vi "Inspect Main.vi"() -> ()   [LabVIEW 2019]
uses:
  Inspect States.ctl
  Common.llb/IVB Global Variable Data Structure.ctl
  Common.llb/IVB Global Variable Type.ctl
  Common.llb/IVB Global Variable Data Type.ctl
  Common.llb/IVB State Machine Data.ctl
  Common.llb/IVB State Machine - States Array.ctl
  Common.llb/IVB State Machine - State.ctl
  Common.llb/IVB State Machine - Transitions Array.ctl
  Common.llb/IVB State Machine - Transition.ctl
  Common.llb/IVB State Machine - Free Labels Array.ctl
  Common.llb/IVB State Machine - Free Label.ctl
  Common.llb/IVB Custom UI - Data.ctl
  Common.llb/IVB Measure ID.ctl
  Common.llb/IVB Execution Function Code.ctl
  Common.llb/IVB VDM Palette Type.ctl
  Common.llb/IVB Decision Maker - Step Results AND Function.ctl
  <vilib>/Utility/sysdir.llb/System Directory Type.ctl
  Common.llb/IVB Results Manager Function.ctl
  Common.llb/IVB CoordSys Manager Function.ctl
  Common.llb/IVB ROI Manager Function.ctl
  Common.llb/IVB State Machine Data Manager Function.ctl
  Common.llb/IVB Palette Manager Function.ctl
  Common.llb/IVB Image Providers Manager Function.ctl
  Common.llb/IVB Global Variable - Manager Mode.ctl
  Common.llb/IVB Custom UI Manager Function.ctl
  Common.llb/IVB Codegen Globals.vi
  Common.llb/IVB Application Paths Global.vi
panel:
  in  "VBAI User Palettes Folder":string="National Instruments\\Vision Builder AI\\Palettes"
  in  "VBAI Flat Field Folder":string="National Instruments\\Vision Builder AI\\Flat Field"
  in  "VBAI Calibration Folder":string="National Instruments\\Vision Builder AI\\Calibration"
  in  "Custom UI Data":T1={"VI Path"=path "", "Use Custom UI"=FALSE, "Show Stats"=TRUE, "Show Table BG Color"=TRUE, "Auto Populate Table"=TRUE, "Table Measure IDs"=[{"Step GUID"="", "Result GUID"="{BE7D05E6-89B2-42AA-A48C-21281F1D1FF2}", "Index"=0}, {"Step GUID"="04378377", "Result GUID"="PASS/FAIL", "Index"=0}, {"Step GUID"="88198009", "Result GUID"="PASS/FAIL", "Index"=0}, {"Step GUID"="03525588", "Result GUID"="PASS/FAIL", "Index"=0}, {"Step GUID"="93671840", "Result GUID"="PASS/FAIL", "Index"=0}, {"Step GUID"="87659981", "Result GUID"="PASS/FAIL", "Index"=0}, {"Step GUID"="92409063", "Result GUID"="PASS/FAIL", "Index"=0}, {"Step GUID"="18845728", "Result GUID"="PASS/FAIL", "Index"=0}, {"Step GUID"="52930538", "Result GUID"="PASS/FAIL", "Index"=0}], "FP Width"=1007, "FP Height"=634, "Version"="6.1.0.0", "Strip Chart Data"={"Names"=[], "History Size"=[]}}
  in  "Inspection Name":string="LICENSE PLATE"
  in  "State Data":T3 {"Transitions"."Scale"."Y" format="%.2f"; "Transitions"."Scale"."X" format="%.2f"}
  out "Image":T10(plugin-control)
  in  "Global Variable Data":T11[](array[typedef])
  in  "Initial State":T14
  in  "Stop":bool
  out "Pass Fail":bool=TRUE caption="Inspection Status"
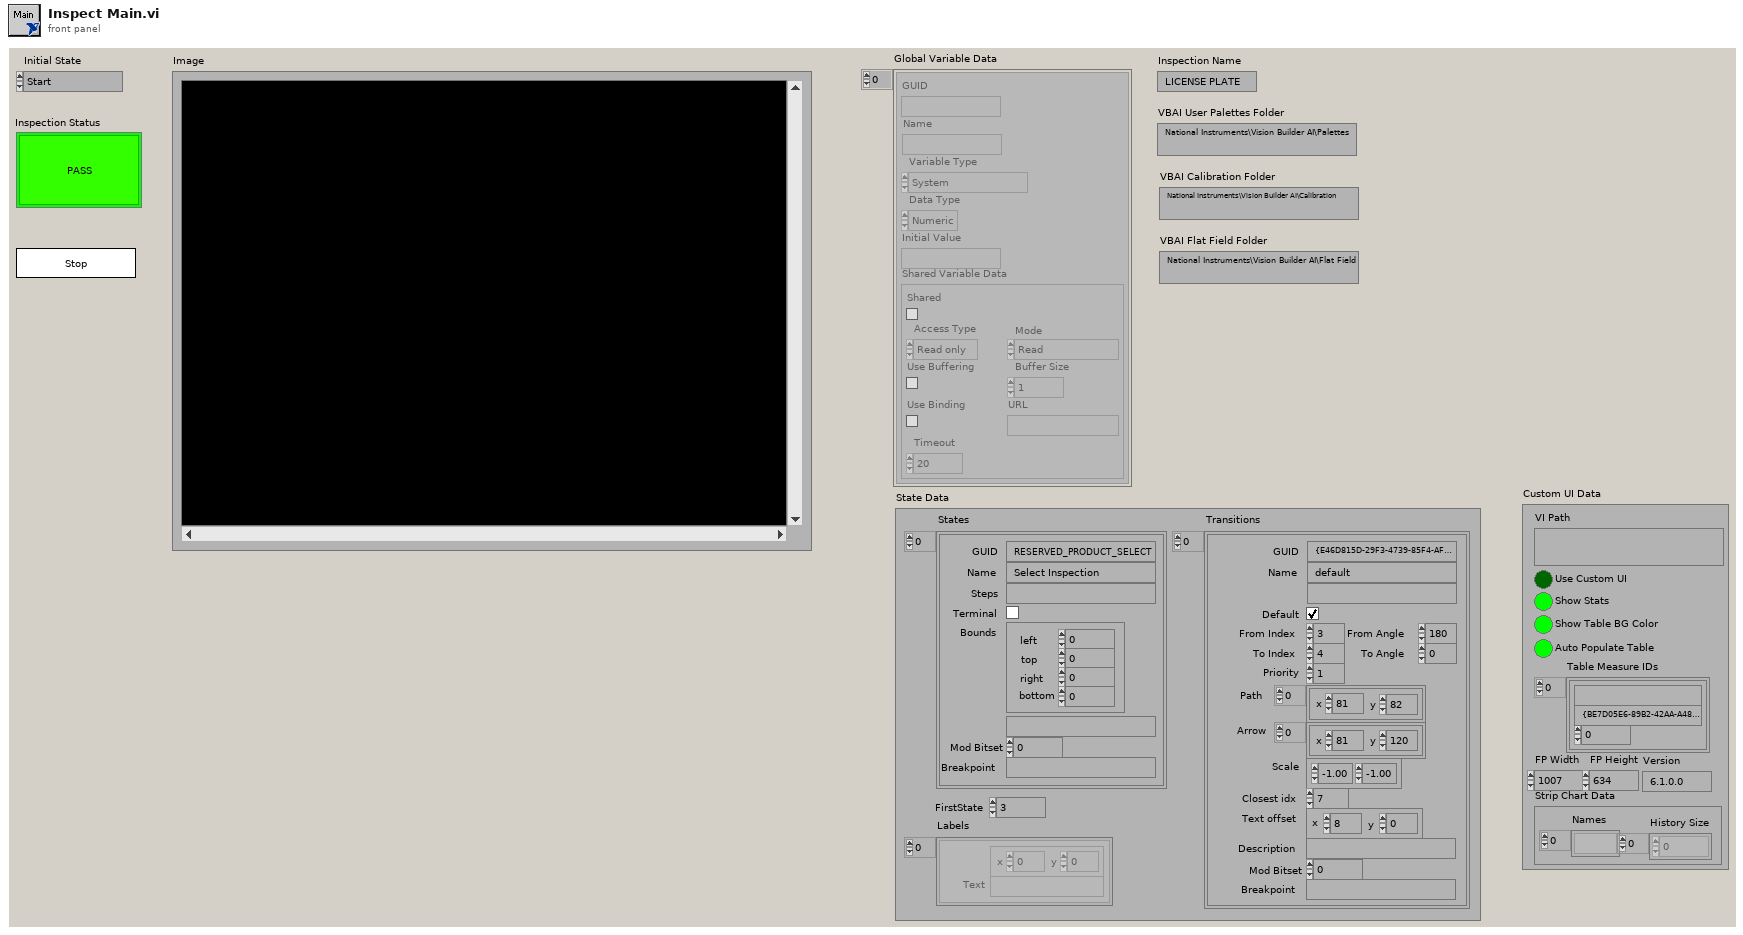
[diagram p1: front panel]
types:
  T1 = typedef "IVB Custom UI - Data.ctl" = cluster{"VI Path":path, "Use Custom UI":bool, "Show Stats":bool, "Show Table BG Color":bool, "Auto Populate Table":bool, "Table Measure IDs":T2[], "FP Width":u32, "FP Height":u32, "Version":string, "Strip Chart Data":cluster{"Names":string[], "History Size":u32[]}}
  T2 = typedef "IVB Measure ID.ctl" = cluster{"Step GUID":string, "Result GUID":string, "Index":i32}
  T3 = typedef "IVB State Machine Data.ctl" = cluster{"States":T4, "Transitions":T6, "FirstState":i32, "Labels":T8}
  T4 = typedef "IVB State Machine - States Array.ctl" = T5[]
  T5 = typedef "IVB State Machine - State.ctl" = cluster{"GUID":string, "Name":string, "Steps":string, "Terminal":bool, "Bounds":cluster{"left":i16, "top":i16, "right":i16, "bottom":i16}, "Description":string, "Mod Bitset":i32, "Breakpoint":string}
  T6 = typedef "IVB State Machine - Transitions Array.ctl" = T7[]
  T7 = typedef "IVB State Machine - Transition.ctl" = cluster{"GUID":string, "Name":string, "Transition Criteria":string, "Default":bool, "From Index":i32, "To Index":i32, "Priority":i32, "Path":cluster{"x":i16, "y":i16}[], "Arrow":cluster{"x":i16, "y":i16}[], "Scale":cluster{"X":dbl, "Y":dbl}, "Closest idx":u16, "Text offset":cluster{"x":i16, "y":i16}, "From Angle":dbl, "To Angle":dbl, "Description":string, "Mod Bitset":i32, "Breakpoint":string}
  T8 = typedef "IVB State Machine - Free Labels Array.ctl" = T9[]
  T9 = typedef "IVB State Machine - Free Label.ctl" = cluster{"Location":cluster{"x":i16, "y":i16}, "Text":string}
  T10 = typedef "IMAQ Image.ctl" = refnum<image>
  T11 = typedef "IVB Global Variable Data Structure.ctl" = cluster{"GUID":string, "Name":string, "Variable Type":T12, "Data Type":T13, "Initial Value":string, "Shared Variable Data":cluster{"Shared":bool, "Access Type":enum16{"Read only", "Write only", "Read/write"}, "Mode":enum16{"Read", "Write", "ReadWrite", "BufferedRead", "BufferedReadWrite"}, "Use Buffering":bool, "Buffer Size":u32, "Use Binding":bool, "URL":string, "Timeout":i32}}
  T12 = typedef "IVB Global Variable Type.ctl" = enum32{"Measurement", "System", "System (User-defined)", "Inspection", "Network", "Custom UI"}
  T13 = typedef "IVB Global Variable Data Type.ctl" = enum16{"Numeric", "Boolean", "String", "Point", "Image", "1D Numeric", "1D Boolean", "1D String"}
  T14 = typedef "Inspect States.ctl" = enum16{"Start", "Inspect", "End"}
  T15 = typedef "IVB VDM Palette Type.ctl" = enum16{"Grayscale", "Binary", "Gradient", "Rainbow", "Temperature", "User Defined", "Binary 16 Bit", "Gradient 16 Bit", "Rainbow 16 Bit", "Temperature 16 Bit", "User Defined 16 Bit"}
  T16 = typedef "IVB Execution Function Code.ctl" = enum16{"Setup", "Exec", "Cleanup"}
  T17 = typedef "IVB Palette Manager Function.ctl" = enum16{"Enumerate Palettes", "Get Palette"}
  T18 = typedef "IVB State Machine Data Manager Function.ctl" = enum16{"Init", "Reset to Default", "Get All", "Set All", "Get State Inspection Steps", "Set State Inspection Steps", "Get State Transition Criteria", "Set State Transition Criteria", "Get Current State", "Set Current State"}
  T19 = typedef "IVB ROI Manager Function.ctl" = enum16{"Initialize", "Reset", "Log ROI", "Get ROI", "Set All ROIs", "Get All ROIs", "Delete ROI"}
  T20 = typedef "IVB CoordSys Manager Function.ctl" = enum16{"Reset", "Log REF CoordSys", "Log NEW CoordSys", "Get Coordsys", "Delete Src", "Get All CoordSys", "Set All CoordSys", "Clear All CoordSys"}
  T21 = typedef "IVB Results Manager Function.ctl" = enum16{"Reset", "Add New Result Source", "Update Results", "Update Only Results", "Clear Results", "Delete Result Source", "Get All Results", "Get Results / Src", "Get Results/Src/Object Index (DO NOT USE ANYMORE)", "Get All Results (Flatten String)", "Put All Results (Flatten String)", "Clear Multiple Results", "Init", "Dispose"}
  T22 = typedef "IVB Global Variable - Manager Mode.ctl" = enum16{"Init", "Delete User Defined", "Update User Defined", "Get All User Defined", "Get All System", "Set Current Value System", "Set Current Value User Defined", "Add/Update Variable"}
  T23 = typedef "IVB Image Providers Manager Function.ctl" = enum16{"Reset", "Register Image Source", "Unregister Source", "Get Image", "Get Image Sources", "Update Image Source"}
  T24 = enum16{"Set User Defined Data", "Get User Defined Data"}
  T25 = typedef "IVB Custom UI Manager Function.ctl" = enum32{"Init", "Get Data", "Reset VI Ref", "Close"}
  T26 = enum32{"Invalid", "Default", "Floating", "Floating/Auto-Hide", "Modal"}
  T27 = enum32{"invalid app kind", "Development System", "Run Time System", "Student Edition", "Embedded LabVIEW", "Evaluation", "Custom"}
  T28 = typedef "System Directory Type.ctl" = i32
  T29 = typedef "IVB Decision Maker - Step Results AND Function.ctl" = enum16{"Reset", "Set Step Result", "Get Step Results AND"}
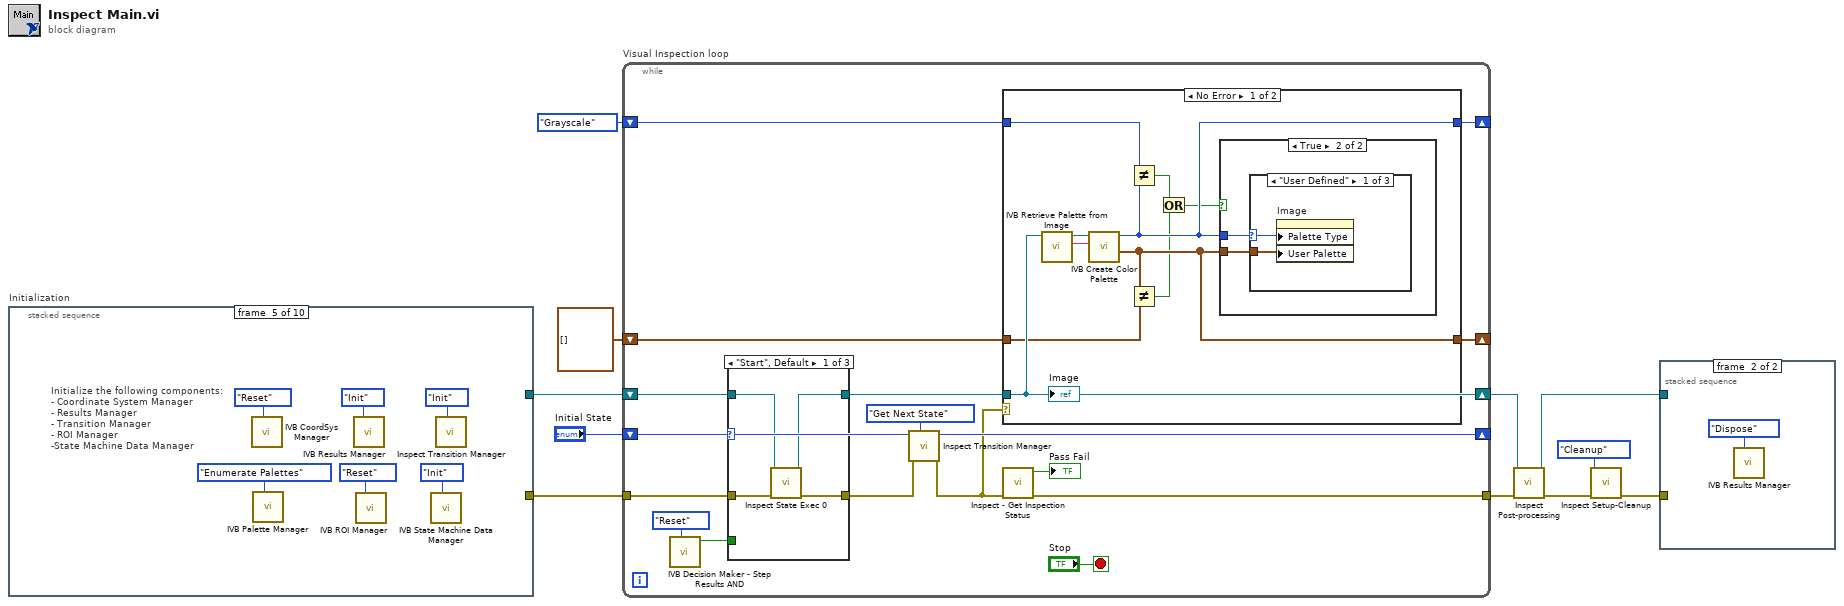
[diagram p0: block diagram]
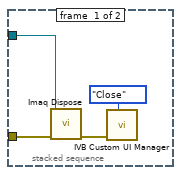
[diagram p2: hidden frame]
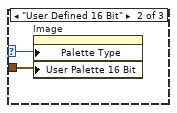
[diagram p4: hidden frame]
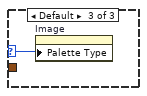
[diagram p5: hidden frame]
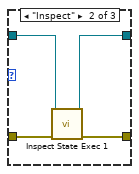
[diagram p7: hidden frame]
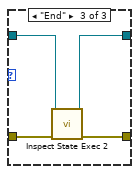
[diagram p8: hidden frame]
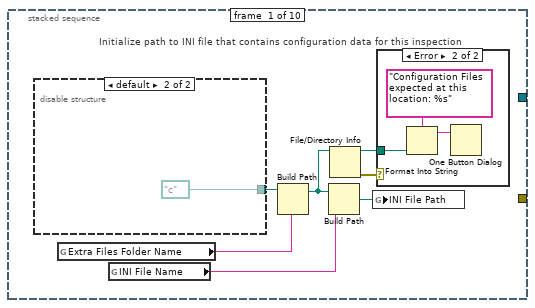
[diagram p9: hidden frame]
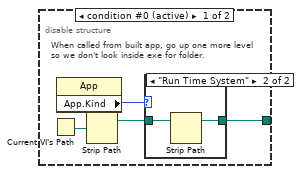
[diagram p11: hidden frame]
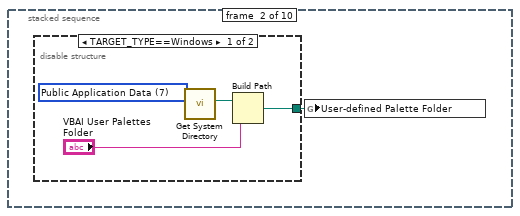
[diagram p13: hidden frame]
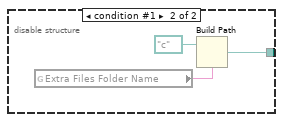
[diagram p14: hidden frame]
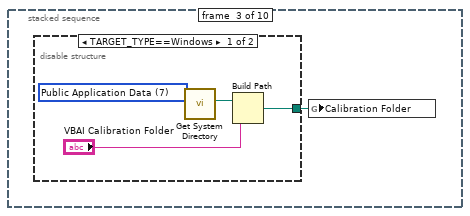
[diagram p15: hidden frame]
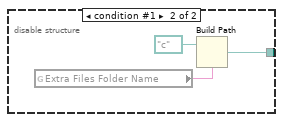
[diagram p16: hidden frame]
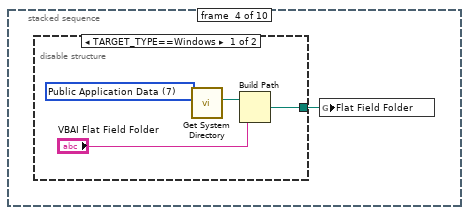
[diagram p17: hidden frame]
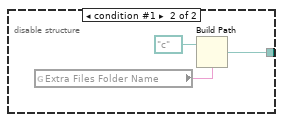
[diagram p18: hidden frame]
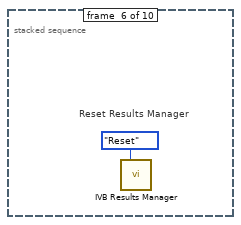
[diagram p19: hidden frame]
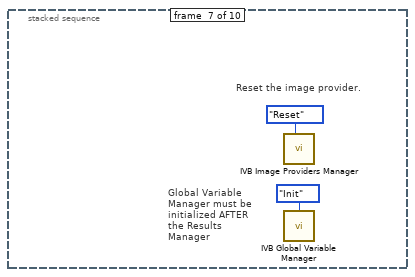
[diagram p20: hidden frame]
diagram:
  n1 = stacked-sequence "Initialization" {
    tunnel: [_ _ _ _ _ _ _ _ _ w81] -> w8
    tunnel: [_ _ _ _ _ _ _ _ _ w80] -> w9
    frame #0 {
      # "Initialize path to INI file that contains configuration data for this inspection"
      n2 = disable-structure shown="default" {
        disable-tunnel: [w22 path "c:/" ("stripped path")] -> w18
        frame condition #0 (active) {
          # "When called from built app, go up one more level so we don't look inside exe for folder."
          n3 = Current VI's Path() -> (path=w25:path)
          n4 = property class="App"() -> ("App.Kind"=w24:T27)  [unwired: 2 in, 2 out]
          n5 = Strip Path(path=w25) -> (stripped path=w23:path)  [unwired: 1 out]
          n6 = case shown="\"Run Time System\"" w24 {
            tunnel: w23 -> [w26 w28]
            tunnel: [w26 w27] -> w22
            frame Default {
            }
            frame "Run Time System" {
              n7 = Strip Path(path=w28) -> (stripped path=w27:path)  [unwired: 1 out]
            }
          }
        }
        frame condition #1 {
        }
      }
      n8 = global read "IVB Codegen Globals.vi" "Extra Files Folder Name"() -> (w17:string)
      n9 = global read "IVB Codegen Globals.vi" "INI File Name"() -> (w16:string)
      n10 = Build Path(base path=w18, name or relative path=w17) -> (appended path=w13:path)
      n11 = Build Path(base path=w13, name or relative path=w16) -> (appended path=w15:path)
      n12 = File/Directory Info(path=w13) -> (path out=w12:path, error out=w14:errorcluster)  [unwired: 1 in, 5 out]
      n13 = global write "IVB Application Paths Global.vi" "INI File Path"(w15) -> ()
      n14 = case shown="Error" w14 {
        tunnel: w12 -> [_ w21]
        frame No Error {
        }
        frame Error {
          n15 = Format Into String(format string="Configuration Files expected at this location: %s", w21) -> (resulting string=w20:string)  [unwired: 2 in, 1 out]
          n16 = One Button Dialog(message=w20) -> ()  [unwired: 1 in, 1 out]
        }
      }
    }
    frame #1 {
      n17 = disable-structure shown="TARGET_TYPE==Windows" {
        disable-tunnel: [w33 w35] -> w30
        frame condition #0 (active) {
          w32 = T28 7 items=["User Home"=0, "User Desktop"=1, "User Documents"=2, "User Application Data"=3, "User Preferences"=4, "User Temporary"=5, "Public Documents"=6, "Public Application Data"=7, "Public Preferences"=8, "Public Cache"=13, "System Core Libraries"=9, "System Installed Libraries"=10, "Application Files"=11, "Boot Volume Root"=12] ("system directory type")
          n18 = call <vilib>:"Get System Directory.vi"("system directory type"=w32) -> ("system directory"=w31:path)  [unwired: 10 in]
          n19 = Build Path(base path=w31, name or relative path="VBAI User Palettes Folder") -> (appended path=w33:path)
        }
        frame condition #1 {
          n20 = global read "IVB Codegen Globals.vi" "Extra Files Folder Name"() -> (w37:string)
          n21 = Build Path(base path=path "c:/" ("stripped path"), name or relative path=w37) -> (appended path=w35:path)
        }
      }
      n22 = global write "IVB Application Paths Global.vi" "User-defined Palette Folder"(w30) -> ()
    }
    frame #2 {
      n23 = disable-structure shown="TARGET_TYPE==Windows" {
        disable-tunnel: [w41 w43] -> w38
        frame condition #0 (active) {
          w40 = T28 7 items=["User Home"=0, "User Desktop"=1, "User Documents"=2, "User Application Data"=3, "User Preferences"=4, "User Temporary"=5, "Public Documents"=6, "Public Application Data"=7, "Public Preferences"=8, "Public Cache"=13, "System Core Libraries"=9, "System Installed Libraries"=10, "Application Files"=11, "Boot Volume Root"=12] ("system directory type")
          n24 = call <vilib>:"Get System Directory.vi"("system directory type"=w40) -> ("system directory"=w39:path)  [unwired: 10 in]
          n25 = Build Path(base path=w39, name or relative path="VBAI Calibration Folder") -> (appended path=w41:path)
        }
        frame condition #1 {
          n26 = global read "IVB Codegen Globals.vi" "Extra Files Folder Name"() -> (w45:string)
          n27 = Build Path(base path=path "c:/" ("stripped path"), name or relative path=w45) -> (appended path=w43:path)
        }
      }
      n28 = global write "IVB Application Paths Global.vi" "Calibration Folder"(w38) -> ()
    }
    frame #3 {
      n29 = disable-structure shown="TARGET_TYPE==Windows" {
        disable-tunnel: [w49 w51] -> w46
        frame condition #0 (active) {
          w48 = T28 7 items=["User Home"=0, "User Desktop"=1, "User Documents"=2, "User Application Data"=3, "User Preferences"=4, "User Temporary"=5, "Public Documents"=6, "Public Application Data"=7, "Public Preferences"=8, "Public Cache"=13, "System Core Libraries"=9, "System Installed Libraries"=10, "Application Files"=11, "Boot Volume Root"=12] ("system directory type")
          n30 = call <vilib>:"Get System Directory.vi"("system directory type"=w48) -> ("system directory"=w47:path)  [unwired: 10 in]
          n31 = Build Path(base path=w47, name or relative path="VBAI Flat Field Folder") -> (appended path=w49:path)
        }
        frame condition #1 {
          n32 = global read "IVB Codegen Globals.vi" "Extra Files Folder Name"() -> (w53:string)
          n33 = Build Path(base path=path "c:/" ("stripped path"), name or relative path=w53) -> (appended path=w51:path)
        }
      }
      n34 = global write "IVB Application Paths Global.vi" "Flat Field Folder"(w46) -> ()
    }
    frame #4 {
      # "Initialize the following components:\n- Coordinate System Manager\n- Results Manager\n- Transition Manager\n- ROI Manager\n-State Machine Data Manager"
      n35 = call "IVB CoordSys Manager.vi"("Function"=IVB_CoordSys_Manager_Function."Reset") -> ()  [unwired: 7 in, 4 out]
      n36 = call "IVB Palette Manager.vi"("Function"=IVB_Palette_Manager_Function."Enumerate Palettes") -> ()  [unwired: 6 in, 5 out]
      n37 = call "IVB Results Manager.vi"("Function"=IVB_Results_Manager_Function."Init") -> ()  [unwired: 10 in, 5 out]
      n38 = call "IVB ROI Manager.vi"("Function"=IVB_ROI_Manager_Function."Reset") -> ()  [unwired: 9 in, 6 out]
      n39 = call "IVB State Machine Data Manager.vi"("Function"=IVB_State_Machine_Data_Manager_Function."Init") -> ()  [unwired: 5 in, 6 out]
      n40 = call "Inspect Transition Manager.vi"("Function"=enum16{"Init", "Get Next State"}."Init" ("Enum")) -> ()  [unwired: 9 in, 2 out]
    }
    frame #5 {
      # "Reset Results Manager"
      n41 = call "IVB Results Manager.vi"("Function"=IVB_Results_Manager_Function."Reset") -> ()  [unwired: 10 in, 5 out]
    }
    frame #6 {
      # "Global Variable Manager must be initialized AFTER the Results Manager"
      # "Reset the image provider."
      n42 = call "IVB Image Providers Manager.vi"("Function"=IVB_Image_Providers_Manager_Function."Reset") -> ()  [unwired: 7 in, 4 out]
      n43 = call "IVB Global Variable Manager.vi"("Function"=IVB_Global_Variable_-_Manager_Mode."Init") -> ()  [unwired: 13 in, 2 out]
    }
    frame #7 {
      # "Initialize global variables."
      n44 = call "IVB State Machine Data Manager.vi"("Function"=IVB_State_Machine_Data_Manager_Function."Set All", "State Data In"="State Data") -> ()  [unwired: 4 in, 6 out]
      n45 = call "Inspect Init Global Variable Values.vi"("Inspection Name"="Inspection Name") -> ()  [unwired: 11 in]
      n46 = call "IVB Global Variable - Set Get All User Defined.vi"("Mode"=T24."Set User Defined Data", "Global Variables in"="Global Variable Data") -> ()  [unwired: 8 in, 2 out]
    }
    frame #8 {
      # "Only useful if using a Custom UI"
      n47 = call "IVB Custom UI Manager.vi"("Mode"=IVB_Custom_UI_Manager_Function."Init", "Settings In"="Custom UI Data") -> ("Cust UI VI Ref"=w68:refnum<vi>, "Settings Out"=w70:T1)  [unwired: 5 in, 3 out]
      n48 = Unbundle By Name(w70) -> ("Use Custom UI"=w69:bool)
      n49 = disable-structure shown="TARGET_TYPE==Windows" {
        disable-tunnel: w69 -> [w74 _]
        disable-tunnel: w68 -> [w73 _]
        frame condition #0 (active) {
          n50 = case shown="True" w74 {
            tunnel: w73 -> [_ w77]
            frame False {
            }
            frame True {
              w76 = TRUE ("Front Panel Window:Open")
              n51 = property class="VI Interface Type 1"(reference=w77, "Front Panel.TitleBarVis"=w76, "Front Panel.Open"=w76, "FP.Behavior"=T26."Floating" ("Front Panel Window:Behavior")) -> ()  [unwired: 1 in, 2 out]
            }
          }
        }
        frame condition #1 {
        }
      }
    }
    frame #9 {
      # "Initialize the visual inspection components\nand run the pre-processing code."
      n52 = call "IMAQ Create"("Image Name"="VBAI Image") -> ("New Image"=w79:T10)  [unwired: 4 in, 1 out]
      n53 = call "Inspect Setup-Cleanup.vi"("Function"=IVB_Execution_Function_Code."Setup") -> ("error out"=w82:errorcluster)  [unwired: 10 in]
      n54 = call "Inspect Pre-processing.vi"("error in (no error)"=w82, "Image Src"=w79) -> ("error out"=w81:errorcluster, "Image Out"=w80:T10)  [unwired: 8 in]
    }
  }
  n55 = while "Visual Inspection loop" {
    tunnel: [w98] -> w7
    tunnel: w8 -> [w99]
    shift-right: [w89] -> w5
    shift-left: w9 -> [w97]
    shift-right: [w95] -> _
    shift-left: "Initial State" -> [w96]
    shift-right: [w85] -> _
    shift-left: IVB_VDM_Palette_Type."Grayscale" ("Palette Type") -> [w84]
    shift-right: [w87] -> _
    shift-left: cluster{"Red":u8, "Green":u8, "Blue":u8}[] [] ("Color Palette") -> [w86]
    stop <- "Stop" stop-if-true
    n56 = call "IVB Decision Maker - Step Results AND.vi"("Function"=IVB_Decision_Maker_-_Step_Results_AND_Function."Reset") -> ("Status"=w90:bool)  [unwired: 10 in]
    n57 = case "Main Case Structure" shown="\"Start\", Default" w96 {
      tunnel: w97 -> [w123 w127 w131]
      tunnel: [w120 w124 w128] -> w93
      tunnel: w99 -> [w122 w126 w130]
      tunnel: [w121 w125 w129] -> w89
      tunnel: w90 -> [_ _ _]
      frame "Start", Default {
        n58 = call "Inspect State Exec 0.vi"("error in (no error)"=w122, "Image Src"=w123) -> ("error out"=w120:errorcluster, "Image Out"=w121:T10)  [unwired: 8 in]
      }
      frame "Inspect" {
        n59 = call "Inspect State Exec 1.vi"("error in (no error)"=w126, "Image Src"=w127) -> ("error out"=w124:errorcluster, "Image Out"=w125:T10)  [unwired: 8 in]
      }
      frame "End" {
        n60 = call "Inspect State Exec 2.vi"("error in (no error)"=w130, "Image Src"=w131) -> ("error out"=w128:errorcluster, "Image Out"=w129:T10)  [unwired: 8 in]
      }
    }
    n61 = call "Inspect Transition Manager.vi"("Function"=enum16{"Init", "Get Next State"}."Get Next State" ("Enum"), "error in (no error)"=w93, "Current State"=w96) -> ("error out"=w88:errorcluster, "Next State"=w95:T14)  [unwired: 7 in]
    n62 = case shown="No Error" w88 {
      tunnel: w89 -> [w108 _]
      tunnel: [w107 w119] -> w87
      tunnel: w86 -> [w106 w119]
      tunnel: [w105 w118] -> w85
      tunnel: w84 -> [w101 w118]
      frame No Error {
        n63 = call "IVB Retrieve Palette from Image.vi"("Image in"=w108) -> ("Palette GUID"=w109:string, "Image out"=w110:T10)  [unwired: 7 in, 2 out]
        n64 = call "IVB Create Color Palette.vi"("Palette GUID in"=w109, "Image"=w110) -> ("Color Palette"=w107:cluster{"Red":u8, "Green":u8, "Blue":u8}[], "Palette Type"=w105:T15)  [unwired: 7 in, 1 out]
        n65 = Not Equal?(x=w101, y=w105) -> (x != y?=w104:bool)
        n66 = Not Equal?(x=w107, y=w106) -> (x != y?=w103:bool)
        n67 = Or(x=w104, y=w103) -> (x .or. y?=w102:bool)
        n68 = case shown="True" w102 {
          tunnel: w107 -> [_ w112]
          tunnel: w105 -> [_ w111]
          frame False {
          }
          frame True {
            n69 = case shown="\"User Defined\"" w111 {
              selector: w111 -> [w114 w116 w117]
              tunnel: w112 -> [w113 w115 _]
              frame "User Defined" {
                n70 = property on="Image" class="ImageControl"("Palette Type"=w114, "User Palette"=w113) -> ()  [unwired: 2 in, 2 out]
              }
              frame "User Defined 16 Bit" {
                n71 = property on="Image" class="ImageControl"("Palette Type"=w116, "User Palette 16 Bit"=w115) -> ()  [unwired: 2 in, 2 out]
              }
              frame Default {
                n72 = property on="Image" class="ImageControl"("Palette Type"=w117) -> ()  [unwired: 2 in, 2 out]
              }
            }
          }
        }
        "Image" <- w108
      }
      frame Error {
      }
    }
    n73 = call "Inspect - Get Inspection Status.vi"("error in (no error)"=w88) -> ("error out"=w98:errorcluster, "Inspection Status"=→"Pass Fail":bool)  [unwired: 9 in]
  }
  n74 = call "Inspect Post-processing.vi"("error in (no error)"=w7, "Image Src"=w5) -> ("error out"=w6:errorcluster, "Image Out"=w4:T10)  [unwired: 8 in]
  n75 = call "Inspect Setup-Cleanup.vi"("error in (no error)"=w6, "Function"=IVB_Execution_Function_Code."Cleanup") -> ("error out"=w3:errorcluster)  [unwired: 9 in]
  n76 = stacked-sequence {
    tunnel: w4 -> [w135 _]
    tunnel: w3 -> [w134 _]
    frame #0 {
      n77 = call "Imaq Dispose"("Image"=w135, "error in (no error)"=w134) -> ("error out"=w133:errorcluster)  [unwired: 4 in]
      n78 = call "IVB Custom UI Manager.vi"("Mode"=IVB_Custom_UI_Manager_Function."Close", "error in"=w133) -> ()  [unwired: 5 in, 5 out]
    }
    frame #1 {
      n79 = call "IVB Results Manager.vi"("Function"=IVB_Results_Manager_Function."Dispose") -> ()  [unwired: 10 in, 5 out]
    }
  }
